vi "EnterCONFIGState.vi"(8 "error in (no error)":errorcluster, 10 "Address":u8, 11 "VISA resource name":refnum<visa-resource-name>) -> (0 "error out":errorcluster, 1 "Raw Response":string, 2 "ConfigState":bool, 3 "VISA resource name out":refnum<visa-resource-name>)   [LabVIEW 2020, in "driver_flodx_ph_probe.lvlib"]
doc: "Enters the CONFIG state to configure the ph probe"
uses:
  <instrlib>/RxnRover/FloDx Ph Probe Driver/driver_flodx_ph_probe.lvlib
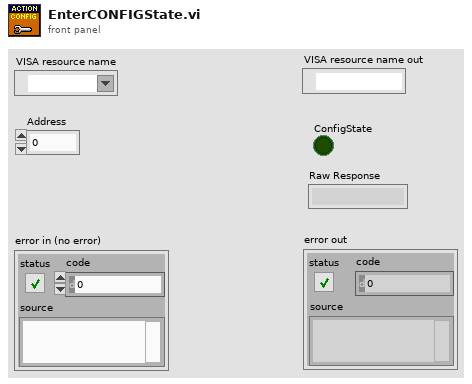
[diagram p1: front panel]
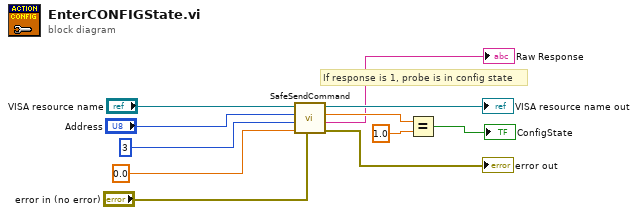
[diagram p0: block diagram]
diagram:
  # "If response is 1, probe is in config state"
  n1 = call <instrlib>:"SafeSendCommand.vi"("error in"="error in (no error)", "Parameter"=sgl 0.0 ("Parameter(float)"), "Command #"=u8 3 ("Command"), "Address #"="Address", "VISA resource name"="VISA resource name") -> ("error out"=→"error out":errorcluster, "Raw Response"=→"Raw Response":string, "Value"=w3:dbl, "VISA resource name out"=→"VISA resource name out":refnum<visa-resource-name>)  [unwired: 3 in]
  n2 = Equal?(x=w3, y=1.0) -> (x = y?=→"ConfigState":bool)
